vi "Init Hardware.vi"(8 "error in (no error)":errorcluster, 11 "DG635 Driver in":refnum<class "DG635 Driver.lvclass">) -> (0 "error out":errorcluster, 3 "DG635 Driver out":refnum<class "DG635 Driver.lvclass">)   [LabVIEW 2021, in "DG635 Driver.lvclass"]
uses:
  DG635 Driver.lvclass
  C:/GitHub/NHMFL_Core/Libraries/Instruments/VISA Instrument/VISA Instrument.lvclass
  VISA Instrument/VISA Instrument.lvclass/VISA Instrument.ctl
  VISA Instrument/Read VISA resource.vi
  VISA Instrument/Write VISA resource.vi
  DG635 Driver.lvclass/DG635 Driver.ctl
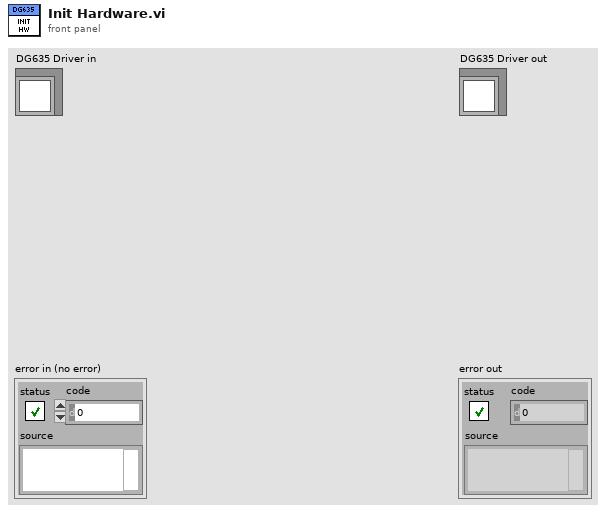
[diagram p1: front panel]
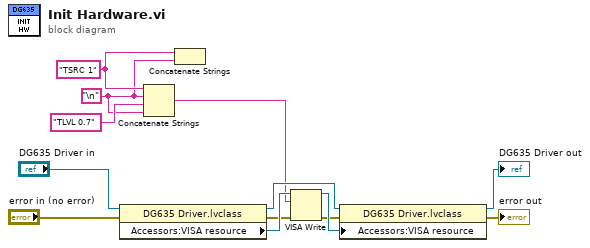
[diagram p0: block diagram]
diagram:
  w2 = "TSRC 1" ("write buffer")
  w1 = "\n"
  n1 = property class="DG635 Driver.lvclass"(reference="DG635 Driver in", error in="error in (no error)") -> (reference out=w12:refnum<class "DG635 Driver.lvclass">, error out=w5:errorcluster, "Accessors:VISA resource"=w8:refnum<visa-resource-name>)
  n2 = Concatenate Strings(w2, w1, "TLVL 0.7" ("write buffer"), w1) -> (w3:string)
  n3 = Concatenate Strings(w2, w1) -> ()  [unwired: 1 out]
  n4 = VISA Write(VISA resource name=w8, write buffer=w3, error in (no error)=w5) -> (VISA resource name out=w7:refnum<visa-resource-name>, error out=w6:errorcluster)  [unwired: 1 out]
  n5 = property class="DG635 Driver.lvclass"(reference=w12, error in=w6, "Accessors:VISA resource"=w7) -> (reference out=→"DG635 Driver out":refnum<class "DG635 Driver.lvclass">, error out=→"error out":errorcluster)
